vi "Periodic Tasks.vi"(8 "error in":errorcluster) -> ()   [LabVIEW 2016]
doc: "This VI runs in parallel to other tasks. It can contain as many user-defined periodic loops as you need. These can carry out PID or other sorts of timed response."
uses:
  <vilib>/Rock Robotics/WPI/Utilities/WPI_GetSetVariantRefNum.vi
  <vilib>/Rock Robotics/Network Tables/NT Write Number.vi
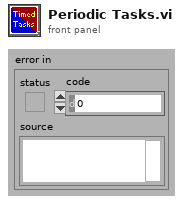
[diagram p1: front panel]
types:
  T1 = typedef "WPI_JoystickDevRef.ctl" = cluster{"Device":T2}
  T2 = typedef "WPI_JoystickDeviceEnum.ctl" = enum16{"USB 0", "USB 1", "USB 2", "USB 3", "USB 4", "USB 5"}
  T3 = typedef "WPI_RobotDriveDevRef.ctl" = cluster{"DevStatus":errorcluster, "Motors[]":T4[], "Square Inputs":bool, "Max Output":dbl}
  T4 = typedef "WPI_MotorControlDeviceRef.ctl" = cluster{"DeviceStatus":errorcluster, "Type":T5, "PWM":cluster{"PWM Channel":T6, "DeadBand":T7}, "CAN":cluster{"Device Number":u8, "SetOutput VI Ref":variant, "GetOutput VI Ref":variant, "Enable VI Ref":variant, "Disable VI Ref":variant, "Data":variant}, "Invert":bool}
  T5 = typedef "WPI_MotorControlType.ctl" = enum16{"PWM", "CAN"}
  T6 = typedef "FPGA_DIOPWMChannel.ctl" = enum8{"PWM 0", "PWM 1", "PWM 2", "PWM 3", "PWM 4", "PWM 5", "PWM 6", "PWM 7", "PWM 8", "PWM 9", "PWM MXP 0", "PWM MXP 1", "PWM MXP 2", "PWM MXP 3", "PWM MXP 4", "PWM MXP 5", "PWM MXP 6", "PWM MXP 7", "PWM MXP 8", "PWM MXP 9", "Invalid"}
  T7 = typedef "WPI_PWMDeadband.ctl" = cluster{"Name":string, "maxPositivePwm":i32, "minPositivePwm":i32, "centerPwm":i32, "maxNegativePwm":i32, "minNegativePwm":i32, "angularRange":u16}
  T8 = cluster{"JoystickDevRef":T1, "RobotDriveDevRef":T3}
  T9 = typedef "WPI_CANTalonSRX_GlobalStatus.ctl" = cluster{"Applied Throttle":dbl, "Module Enabled":bool, "CAN Error":errorcluster, "Closed Loop Error":dbl, "Forward Limit Switch Closed":bool, "Reverse Limit Switch Closed":bool, "Sensor Position":dbl, "Sensor Velocity":dbl, "Current":dbl, "Sticky Fault - Over Temp":bool, "Sticky Fault - Under Voltage":bool, "Sticky Fault - Forward Limit":bool, "Sticky Fault - Reverse Limit":bool, "Sticky Fault - Forward Soft Limit":bool, "Sticky Fault - Reverse Soft Limit":bool, "Brake is Enabled":bool, "Encoder Position":dbl, "Encoder Velocity":dbl, "Encoder Index Count":dbl, "Encoder A Pin State":bool, "Encoder B Pin State":bool, "Encoder Index Pin State":bool, "Analog In":dbl, "Analog In Velocity":dbl, "Temperature (C)":dbl, "Battery Voltage":dbl, "Control 5 Is Supported":bool, "Current Profile Slot Select":dbl, "Pos Div 8":bool, "Vel Div 4":bool, "Pulse Width Position":i32, "Pulse Width Velocity":i32, "Pulse Width Rise To Rise (us)":i32, "Pulse Width Rise To Fall (us)":i32, "Mot Prof Active Is Under Run":bool, "Mot Prof Active Has Under Run":bool, "Mot Prof Active Is Last":bool, "Mot Prof Active Velocity Only":bool, "Mot Prof Active Is Valid":bool, "Mot Prof Buffer Is Full":bool, "Mot Prof Active Profile Slot Select":i32, "Mot Prof NextID":i32, "Mot Prof Count":i32, "Mot Prof Active Velocity":dbl, "Mot Prof Active Position":dbl, "Mot Prof Output Enable":i32}
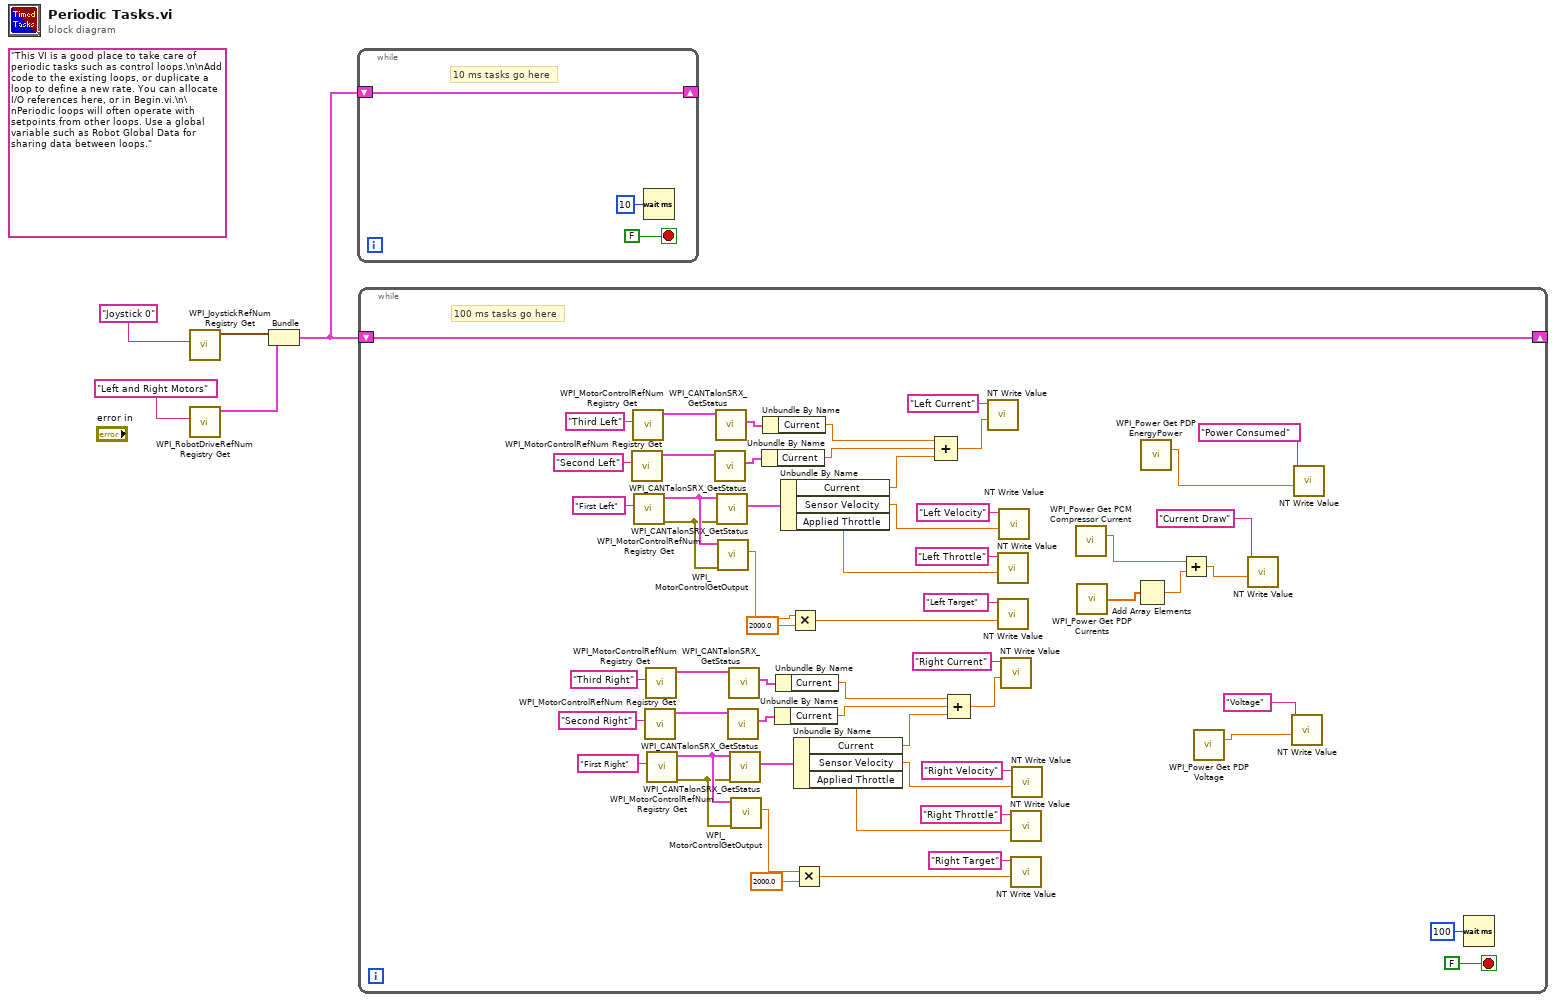
[diagram p0: block diagram]
diagram:
  (unwired) "This VI is a good place to take care of periodic tasks such as control loops.\n\nAdd code to the existing loops, or duplicate a loop to define a new rate. You can allocate I/O references here, or in Begin.vi.\n\nPeriodic loops will often operate with setpoints from other loops. Use a global variable such as Robot Global Data for sharing data between loops."
  n1 = call <vilib>:"WPI_JoystickRefNum Registry Get.vi"("refnum name"="Joystick 0") -> ("JoystickDevRef"=w3:T1)  [unwired: 1 in, 9 out]
  n2 = call <vilib>:"WPI_RobotDriveRefNum Registry Get.vi"("refnum name"="Left and Right Motors") -> ("RobotDriveDevRef"=w2:T3)  [unwired: 1 in, 9 out]
  n3 = Bundle("JoystickDevRef"=w3, "RobotDriveDevRef"=w2) -> (w1:T8)  [unwired: 1 out]
  n4 = while {
    shift-right: [w6] -> _
    shift-left: w1 -> [w6]
    stop <- FALSE stop-if-true
    # "10 ms tasks go here"
    n5 = Wait (ms)(milliseconds to wait=u32 10) -> ()  [unwired: 1 out]
  }
  n6 = while {
    shift-right: [w64] -> _
    shift-left: w1 -> [w64]
    stop <- FALSE stop-if-true
    # "100 ms tasks go here"
    n7 = call <vilib>:"WPI_MotorControlRefNum Registry Get.vi"("refnum name"="Second Left") -> ("MotorControlDevRef"=w34:T4)  [unwired: 9 in, 1 out]
    n8 = call <vilib>:"WPI_MotorControlRefNum Registry Get.vi"("refnum name"="Third Left") -> ("MotorControlDevRef"=w36:T4)  [unwired: 9 in, 1 out]
    n9 = call <vilib>:"WPI_MotorControlRefNum Registry Get.vi"("refnum name"="First Left") -> ("error out"=w25:errorcluster, "MotorControlDevRef"=w26:T4)  [unwired: 9 in]
    n10 = call <vilib>:"WPI_MotorControlRefNum Registry Get.vi"("refnum name"="Second Right") -> ("MotorControlDevRef"=w54:T4)  [unwired: 9 in, 1 out]
    n11 = call <vilib>:"WPI_MotorControlRefNum Registry Get.vi"("refnum name"="Third Right") -> ("MotorControlDevRef"=w56:T4)  [unwired: 9 in, 1 out]
    n12 = call <vilib>:"WPI_MotorControlRefNum Registry Get.vi"("refnum name"="First Right") -> ("error out"=w45:errorcluster, "MotorControlDevRef"=w46:T4)  [unwired: 9 in]
    n13 = call <vilib>:"WPI_CANTalonSRX_GetStatus.vi"("CAN Talon SRX Ref"=w34) -> ("Talon SRX Status"=w37:T9)  [unwired: 8 in, 2 out]
    n14 = call <vilib>:"WPI_CANTalonSRX_GetStatus.vi"("CAN Talon SRX Ref"=w36) -> ("Talon SRX Status"=w38:T9)  [unwired: 8 in, 2 out]
    n15 = call <vilib>:"WPI_CANTalonSRX_GetStatus.vi"("error in (no error)"=w25, "CAN Talon SRX Ref"=w26) -> ("Talon SRX Status"=w27:T9)  [unwired: 7 in, 2 out]
    n16 = call <vilib>:"WPI_MotorControlGetOutput.vi"("error in"=w25, "MotorControlDevRef"=w26) -> ("Output"=w13:dbl)  [unwired: 7 in, 2 out]
    n17 = call <vilib>:"WPI_CANTalonSRX_GetStatus.vi"("CAN Talon SRX Ref"=w54) -> ("Talon SRX Status"=w57:T9)  [unwired: 8 in, 2 out]
    n18 = call <vilib>:"WPI_CANTalonSRX_GetStatus.vi"("CAN Talon SRX Ref"=w56) -> ("Talon SRX Status"=w58:T9)  [unwired: 8 in, 2 out]
    n19 = call <vilib>:"WPI_CANTalonSRX_GetStatus.vi"("error in (no error)"=w45, "CAN Talon SRX Ref"=w46) -> ("Talon SRX Status"=w47:T9)  [unwired: 7 in, 2 out]
    n20 = call <vilib>:"WPI_MotorControlGetOutput.vi"("error in"=w45, "MotorControlDevRef"=w46) -> ("Output"=w15:dbl)  [unwired: 7 in, 2 out]
    n21 = Unbundle By Name(w37) -> ("Current"=w40:dbl)
    n22 = Unbundle By Name(w38) -> ("Current"=w41:dbl)
    n23 = Unbundle By Name(w57) -> ("Current"=w60:dbl)
    n24 = Unbundle By Name(w58) -> ("Current"=w61:dbl)
    n25 = Unbundle By Name(w27) -> ("Current"=w42:dbl, "Sensor Velocity"=w32:dbl, "Applied Throttle"=w39:dbl)
    n26 = Multiply(x=w13, y=2000.0) -> (x*y=w11:dbl)
    n27 = Unbundle By Name(w47) -> ("Current"=w62:dbl, "Sensor Velocity"=w52:dbl, "Applied Throttle"=w59:dbl)
    n28 = Multiply(x=w15, y=2000.0) -> (x*y=w10:dbl)
    n29 = Compound Arithmetic op=ADD(w41, w40, w42) -> (w43:dbl)
    n30 = Compound Arithmetic op=ADD(w61, w60, w62) -> (w63:dbl)
    n31 = call-poly <vilib>:"NT Write Value.vi"("Numeric"=w43, "Name"="Left Current") -> ()  [unwired: 9 in, 1 out]
    n32 = call-poly <vilib>:"NT Write Value.vi"("Numeric"=w39, "Name"="Left Throttle") -> ()  [unwired: 9 in, 1 out]
    n33 = call-poly <vilib>:"NT Write Value.vi"("Numeric"=w11, "Name"="Left Target") -> ()  [unwired: 9 in, 1 out]
    n34 = call-poly <vilib>:"NT Write Value.vi"("Numeric"=w32, "Name"="Left Velocity") -> ()  [unwired: 9 in, 1 out]
    n35 = call-poly <vilib>:"NT Write Value.vi"("Numeric"=w63, "Name"="Right Current") -> ()  [unwired: 9 in, 1 out]
    n36 = call-poly <vilib>:"NT Write Value.vi"("Numeric"=w59, "Name"="Right Throttle") -> ()  [unwired: 9 in, 1 out]
    n37 = call-poly <vilib>:"NT Write Value.vi"("Numeric"=w10, "Name"="Right Target") -> ()  [unwired: 9 in, 1 out]
    n38 = call-poly <vilib>:"NT Write Value.vi"("Numeric"=w52, "Name"="Right Velocity") -> ()  [unwired: 9 in, 1 out]
    n39 = call <vilib>:"WPI_Power Get PCM Compressor Current.vi"() -> ("current (A)"=w22:dbl)  [unwired: 14 in, 1 out]
    n40 = call <vilib>:"WPI_Power Get PDP Currents.vi"() -> ("all currents (A)"=w20:dbl[])  [unwired: 13 in, 2 out]
    n41 = Add Array Elements(numeric array=w20) -> (sum=w21:dbl)
    n42 = call <vilib>:"WPI_Power Get PDP EnergyPower.vi"() -> ("Energy (J)"=w9:dbl)  [unwired: 13 in, 2 out]
    n43 = Add(x=w22, y=w21) -> (x+y=w23:dbl)
    n44 = call <vilib>:"WPI_Power Get PDP Voltage.vi"() -> ("voltage (V)"=w17:dbl)  [unwired: 14 in, 1 out]
    n45 = call-poly <vilib>:"NT Write Value.vi"("Numeric"=w23, "Name"="Current Draw") -> ()  [unwired: 9 in, 1 out]
    n46 = call-poly <vilib>:"NT Write Value.vi"("Numeric"=w17, "Name"="Voltage") -> ()  [unwired: 9 in, 1 out]
    n47 = call-poly <vilib>:"NT Write Value.vi"("Numeric"=w9, "Name"="Power Consumed") -> ()  [unwired: 9 in, 1 out]
    n48 = Wait (ms)(milliseconds to wait=u32 100) -> ()  [unwired: 1 out]
  }
